vi "Test 1.vi"() -> ()   [LabVIEW 2014]
uses:
  <vilib>/Aledyne-TSXperts/Arduino Compatible Compiler for LabVIEW/addons/Complex Numbers/Complex Numbers.lvlib
panel:
  out "result 2":string
  out "Error Out":errorcluster
  in  "Error In":errorcluster
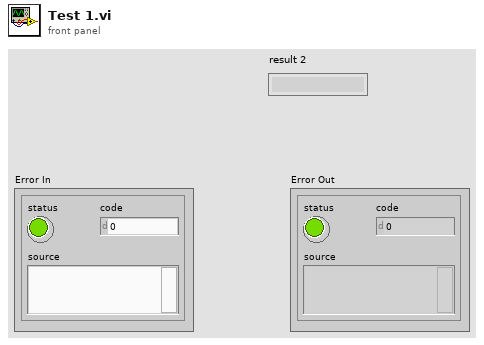
[diagram p1: front panel]
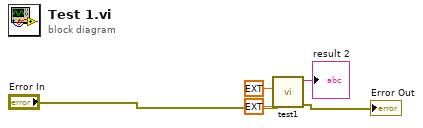
[diagram p0: block diagram]
diagram:
  n1 = call <vilib>:"test1.vi"("error in (no error)"="Error In", "a"=ext 1.0, "nejakaMacZeVraj"=ext 2.0) -> ("error out"=→"Error Out":errorcluster, "result"=→"result 2":string)  [unwired: 7 in]
